vi "Read Address.vi"(8 "error in":errorcluster, 11 "TCP master in":refnum<class "TCP Master.lvclass">) -> (0 "error out":errorcluster, 2 "Address":string, 3 "TCP master out":refnum<class "TCP Master.lvclass">)   [LabVIEW 2021, in "TCP Master.lvclass"]
doc: "Property accessor for the TCP address."
uses:
  TCP Master.lvclass
  TCP Master.lvclass/TCP Master.ctl
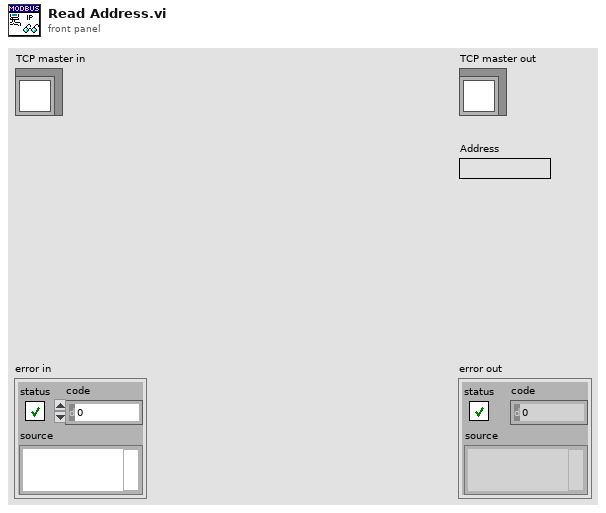
[diagram p1: front panel]
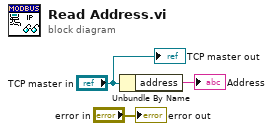
[diagram p0: block diagram]
diagram:
  n1 = Unbundle By Name("TCP master in") -> ("address"=→"Address":string)
  "error out" <- "error in"
  "TCP master out" <- "TCP master in"
